vi "vr.vi"(11 "error in (no error)":errorcluster) -> ()   [LabVIEW 2013]
uses:
  Robot Global Data.vi
panel:
  out "value 2":T1(array[cluster])
  out "Connected 2":bool
  out "Outside loop":i32
  out "Connected":bool
  out "Numeric":i32
  out "value":T2(array[cluster])
  # "e"
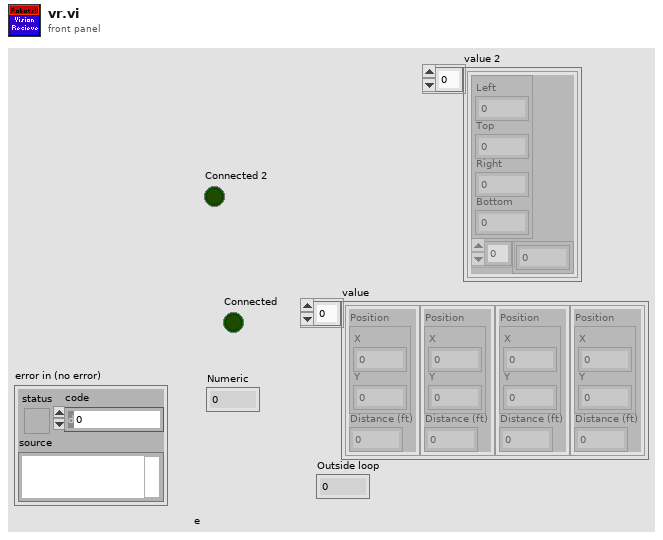
[diagram p1: front panel]
types:
  T1 = cluster{cluster{"Left":dbl, "Top":dbl, "Right":dbl, "Bottom":dbl}, dbl[]}[]
  T2 = cluster{"Position":cluster{"X":dbl, "Y":dbl}, "Distance (ft)":dbl}[]
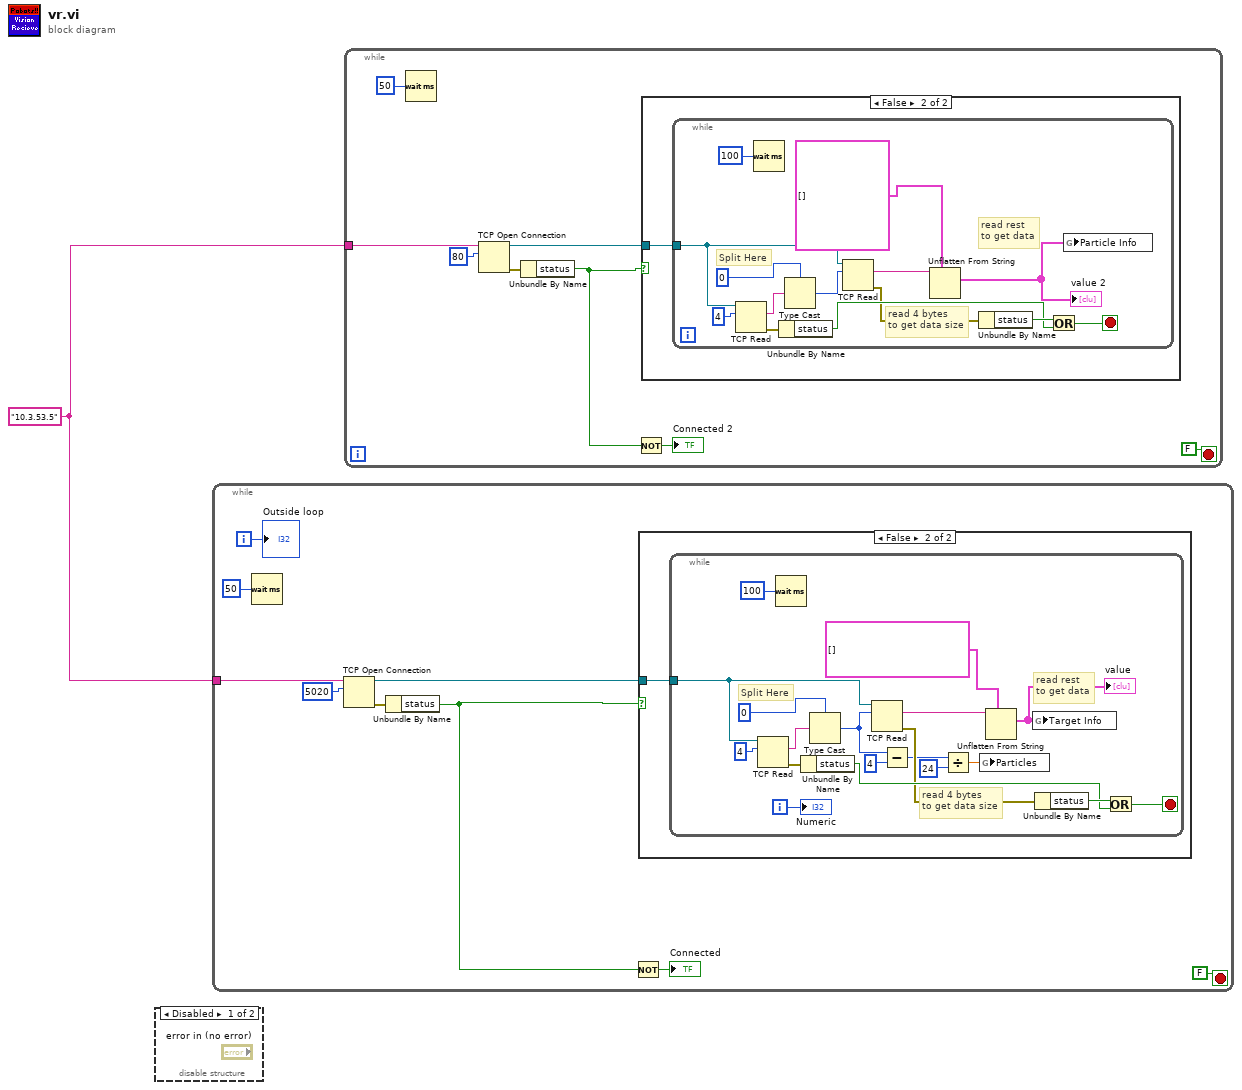
[diagram p0: block diagram]
diagram:
  w1 = "10.3.53.5" ("address")
  n1 = disable-structure shown="Disabled" {
    frame Disabled {
    }
    frame Enabled {
    }
  }
  n2 = while {
    tunnel: w1 -> [w3]
    i -> [w6]
    stop <- FALSE stop-if-true
    n3 = Wait (ms)(milliseconds to wait=u32 50) -> ()  [unwired: 1 out]
    n4 = TCP Open Connection(address=w3, remote port or service name=u16 5020 ("port")) -> (connection ID=w9:refnum<k5>, error out=w10:errorcluster)  [unwired: 3 in]
    n5 = Unbundle By Name(w10) -> ("status"=w2:bool)
    n6 = Not(x=w2) -> (.not. x?=→"Connected":bool)
    n7 = case shown="False" w2 {
      tunnel: w9 -> [_ w11]
      frame True {
      }
      frame False {
        n8 = while {
          tunnel: w11 -> [w30]
          i -> [w19]
          stop <- w21 stop-if-true
          # "Split Here"
          # "read rest\nto get data"
          # "read 4 bytes\nto get data size"
          n9 = TCP Read(connection ID=w30, bytes to read=4) -> (data out=w27:string, error out=w24:errorcluster)  [unwired: 3 in, 1 out]
          n10 = Wait (ms)(milliseconds to wait=u32 100) -> ()  [unwired: 1 out]
          n11 = Unbundle By Name(w24) -> ("status"=w22:bool)
          n12 = Type Cast(type=0, x=w27) -> (*(type *) &x=w16:i32)
          n13 = TCP Read(connection ID=w30, bytes to read=w16) -> (data out=w25:string, error out=w18:errorcluster)  [unwired: 3 in, 1 out]
          n14 = Subtract(x=w16, y=4) -> (x-y=w14:i32)
          n15 = Divide(x=w14, y=24) -> (x/y=w12:dbl)
          n16 = global write "Robot Global Data.vi" "Particles"(w12) -> ()
          n17 = Unflatten From String(type=T2 [], binary string=w25) -> (value=w17:T2)  [unwired: 3 in, 2 out]
          "value" <- w17
          n18 = global write "Robot Global Data.vi" "Target Info"(w17) -> ()
          n19 = Unbundle By Name(w18) -> ("status"=w23:bool)
          n20 = Or(x=w23, y=w22) -> (x .or. y?=w21:bool)
          "Numeric" <- w19
        }
      }
    }
    "Outside loop" <- w6
  }
  n21 = while {
    tunnel: w1 -> [w33]
    stop <- FALSE stop-if-true
    n22 = Wait (ms)(milliseconds to wait=u32 50) -> ()  [unwired: 1 out]
    n23 = TCP Open Connection(address=w33, remote port or service name=u16 80 ("port")) -> (connection ID=w32:refnum<k5>, error out=w38:errorcluster)  [unwired: 3 in]
    n24 = Unbundle By Name(w38) -> ("status"=w31:bool)
    n25 = Not(x=w31) -> (.not. x?=→"Connected 2":bool)
    n26 = case shown="False" w31 {
      tunnel: w32 -> [_ w39]
      frame True {
      }
      frame False {
        n27 = while {
          tunnel: w39 -> [w53]
          stop <- w45 stop-if-true
          # "Split Here"
          # "read rest\nto get data"
          # "read 4 bytes\nto get data size"
          n28 = TCP Read(connection ID=w53, bytes to read=4) -> (data out=w51:string, error out=w48:errorcluster)  [unwired: 3 in, 1 out]
          n29 = Wait (ms)(milliseconds to wait=u32 100) -> ()  [unwired: 1 out]
          n30 = Unbundle By Name(w48) -> ("status"=w46:bool)
          n31 = Type Cast(type=0, x=w51) -> (*(type *) &x=w42:i32)
          n32 = TCP Read(connection ID=w53, bytes to read=w42) -> (data out=w49:string, error out=w43:errorcluster)  [unwired: 3 in, 1 out]
          n33 = Unflatten From String(type=T1 [] ("Scored Particle Info"), binary string=w49) -> (value=w40:T1)  [unwired: 3 in, 2 out]
          "value 2" <- w40
          n34 = Unbundle By Name(w43) -> ("status"=w47:bool)
          n35 = Or(x=w47, y=w46) -> (x .or. y?=w45:bool)
          n36 = global write "Robot Global Data.vi" "Particle Info"(w40) -> ()
        }
      }
    }
  }
